vi "实验4_5.vi"() -> ()   [LabVIEW 2018]
panel:
  out "2D Picture":picture
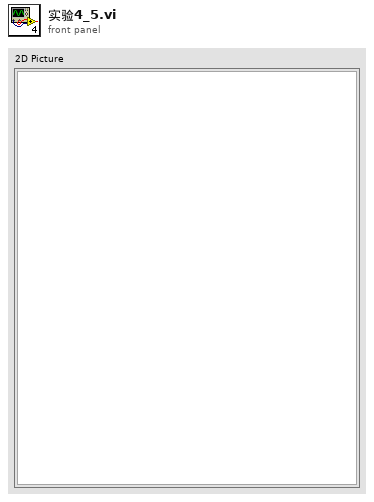
[diagram p1: front panel]
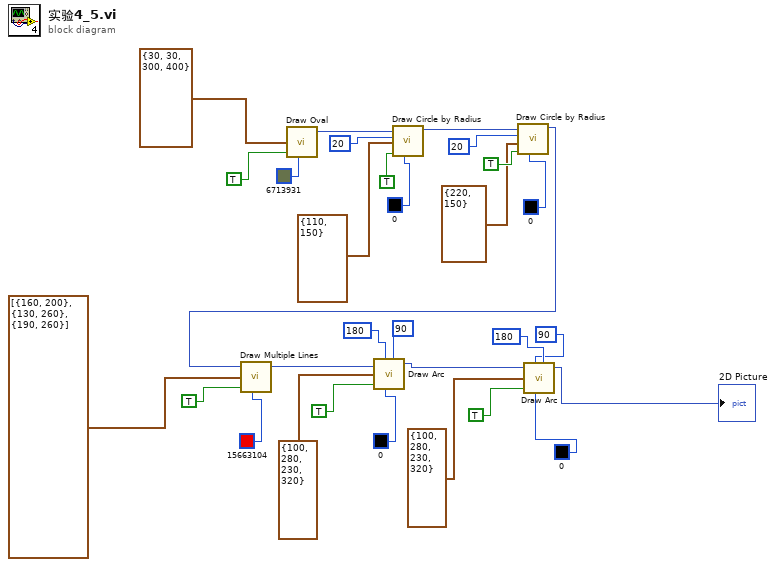
[diagram p0: block diagram]
diagram:
  n1 = call <vilib>:"Draw Oval.vi"("rect"=cluster{i32, i32, i32, i32} {30, 30, 300, 400}, "fill?(F)"=TRUE, "color(black)"=u32 6713931) -> ("new picture"=w27:picture)  [unwired: 6 in]
  n2 = call <vilib>:"Draw Circle by Radius.vi"("color(black)"=u32 0, "fill?(F)"=TRUE, "pixel center"=cluster{i32, i32} {110, 150}, "radius"=20, "picture"=w27) -> ("new picture"=w22:picture)  [unwired: 6 in]
  n3 = call <vilib>:"Draw Circle by Radius.vi"("color(black)"=u32 0, "fill?(F)"=TRUE, "pixel center"=cluster{i32, i32} {220, 150}, "radius"=20, "picture"=w22) -> ("new picture"=w15:picture)  [unwired: 6 in]
  n4 = call <vilib>:"Draw Multiple Lines.vi"("picture"=w15, "line endpoints"=cluster{i32, i32}[] [{160, 200}, {130, 260}, {190, 260}], "fill?(F)"=TRUE, "color(black)"=u32 15663104) -> ("new picture"=w10:picture)  [unwired: 5 in]
  n5 = call <vilib>:"Draw Arc.vi"("picture"=w10, "start angle[degrees]"=180, "rect"=cluster{i32, i32, i32, i32} {100, 280, 230, 320}, "fill?(F)"=TRUE, "color(black)"=u32 0, "arc size[degrees]"=90) -> ("new picture"=w9:picture)  [unwired: 3 in]
  n6 = call <vilib>:"Draw Arc.vi"("picture"=w9, "start angle[degrees]"=90, "rect"=cluster{i32, i32, i32, i32} {100, 280, 230, 320}, "fill?(F)"=TRUE, "color(black)"=u32 0, "arc size[degrees]"=180) -> ("new picture"=→"2D Picture":picture)  [unwired: 3 in]
